vi "CHS_TRAJ_ABS_ODOM_BEGIN.vi"(8 "error in (no error)":errorcluster, 9 "Initial Pose":T1 {"ROTATION"."SIN" format="%13.4f"; "ROTATION"."COS" format="%13.4f"; "ROTATION"."VALUE" format="%13.4f"; "TRANSLATION"."Y" format="%14.3f"; "TRANSLATION"."X" format="%14.3f"}, 10 "Initial Gyro Angle":T3 {"SIN" format="%13.4f"; "COS" format="%13.4f"; "VALUE" format="%13.4f"}) -> (0 "error out":errorcluster)   [LabVIEW 2019]
uses:
  <vilib>/Rock Robotics/WPI/ThirdParty/JAS_Junk/TrajLib/Trajectory_Library.lvlib
  CHS_TRAJECTORY_GLOBALS.vi
  <vilib>/Rock Robotics/WPI/ThirdParty/JAS_Junk/TrajLib/TypeDef/ROTATION2D.ctl
  <vilib>/Rock Robotics/WPI/ThirdParty/JAS_Junk/TrajLib/TypeDef/TRANSLATION2D.ctl
  <vilib>/Rock Robotics/WPI/ThirdParty/JAS_Junk/TrajLib/TypeDef/POSE2D.ctl
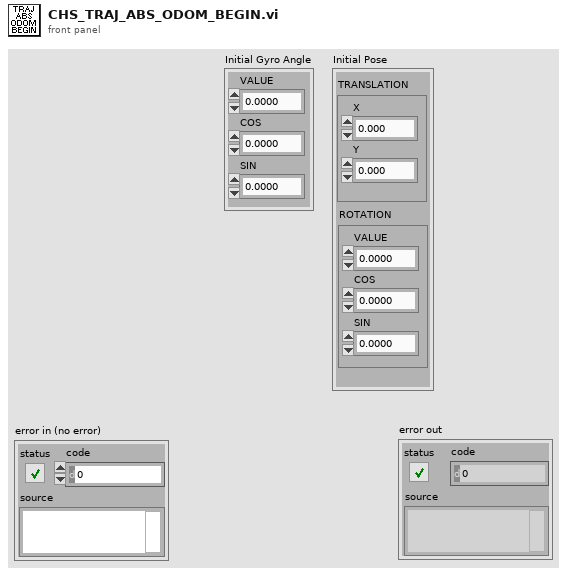
[diagram p1: front panel]
types:
  T1 = typedef "Trajectory_Library.lvlib/POSE2D.ctl" = cluster{"TRANSLATION":T2, "ROTATION":T3}
  T2 = typedef "Trajectory_Library.lvlib/TRANSLATION2D.ctl" = cluster{"X":dbl, "Y":dbl}
  T3 = typedef "Trajectory_Library.lvlib/ROTATION2D.ctl" = cluster{"VALUE":dbl, "COS":dbl, "SIN":dbl}
  T4 = typedef "Trajectory_Library.lvlib/SWERVE_DRIVE_MODULE_POSITION.ctl" = cluster{"Distance":dbl, "Angle":T3, "P":bool}
  T5 = typedef "Trajectory_Library.lvlib/SWERVE_DRIVE_ODOMETRY.ctl" = cluster{"POSE":T1, "GyroOffset":T3, "PreviousAngle":T3, "PrevModulePositions":T4[], "NumModules":i32}
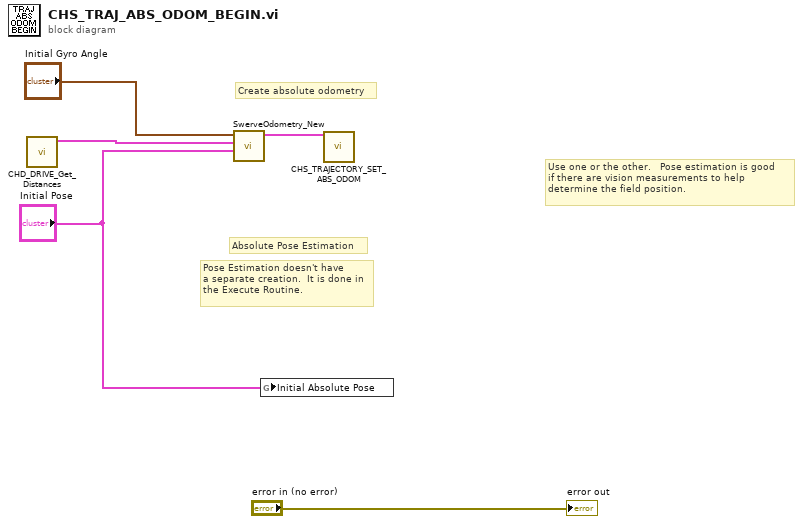
[diagram p0: block diagram]
diagram:
  # "Create absolute odometry"
  # "Absolute Pose Estimation"
  # "Pose Estimation doesn't have\na separate creation.  It is done in\nthe Execute Routine."
  # "Use one or the other.   Pose estimation is good\nif there are vision measurements to help\ndetermine the field position."
  n1 = call "CHD_DRIVE_Get_Distances.vi"() -> ("Swerve Module Positions"=w3:T4[])  [unwired: 11 in]
  n2 = call <vilib>:"SwerveOdometry_New.vi"("InitialPose"="Initial Pose", "Module Positions"=w3, "gyroAngle"="Initial Gyro Angle") -> ("SWERVE_DRIVE_ODOMETRY"=w1:T5)  [unwired: 8 in]
  n3 = global write "CHS_TRAJECTORY_GLOBALS.vi" "Initial Absolute Pose"("Initial Pose") -> ()
  n4 = call "CHS_TRAJECTORY_SET_ABS_ODOM.vi"("Absolue Odometry"=w1) -> ()  [unwired: 11 in]
  "error out" <- "error in (no error)"
